vi "Logger_SARAH.vi"() -> ()   [LabVIEW 2017]
uses:
  DefDeType/ListeMachineEtats.ctl
  DefDeType/ClusterRefCtrlUSBB.ctl
  DefDeType/WhichPath.ctl
  <vilib>/DAQmx/write.llb/DAQmx Write (Digital Bool 1Line 1Point).vi
  <vilib>/DAQmx/read.llb/DAQmx Read (Analog 1D Wfm NChan NSamp).vi
  <vilib>/DAQmx/create/channels.llb/DAQmx Create Channel (DO-Digital Output).vi
  <vilib>/DAQmx/miscellaneous.llb/DAQmx Fill In Error Info.vi
  <vilib>/DAQmx/configure/task.llb/DAQmx Configure Logging (TDMS).vi
  <vilib>/DAQmx/configure/trigger.llb/DAQmx Start Trigger (Digital Edge).vi
panel:
  in  "Tempo Mes-Largage (ms)":i32=1000
  in  "Tempo Houle - Mes (ms)":i32=5000
  in  "Reprocess":bool
  in  "Calibration":bool
  in  "NextTest Num":u32
  out "num iteration":i32
  out "Acquisition Time":dbl(slide) max=10.0 scale=0.0..1000.0
  in  "ModifConfig":bool
  out "Test List":i32(listbox)=-1
  in  "Bouton Stop":bool
  in  "Bouton Rec":bool
  out "Projet :":string
  out "message":string
  in  "Bouton Quit":bool
  out "LoopTime":u32(graph)
  out "Graph1":waveform(dbl)[](graph)
  # "Data Logger"
  # "Actions"
  # "Project"
  # "PCI Channels"
  # "Test List"
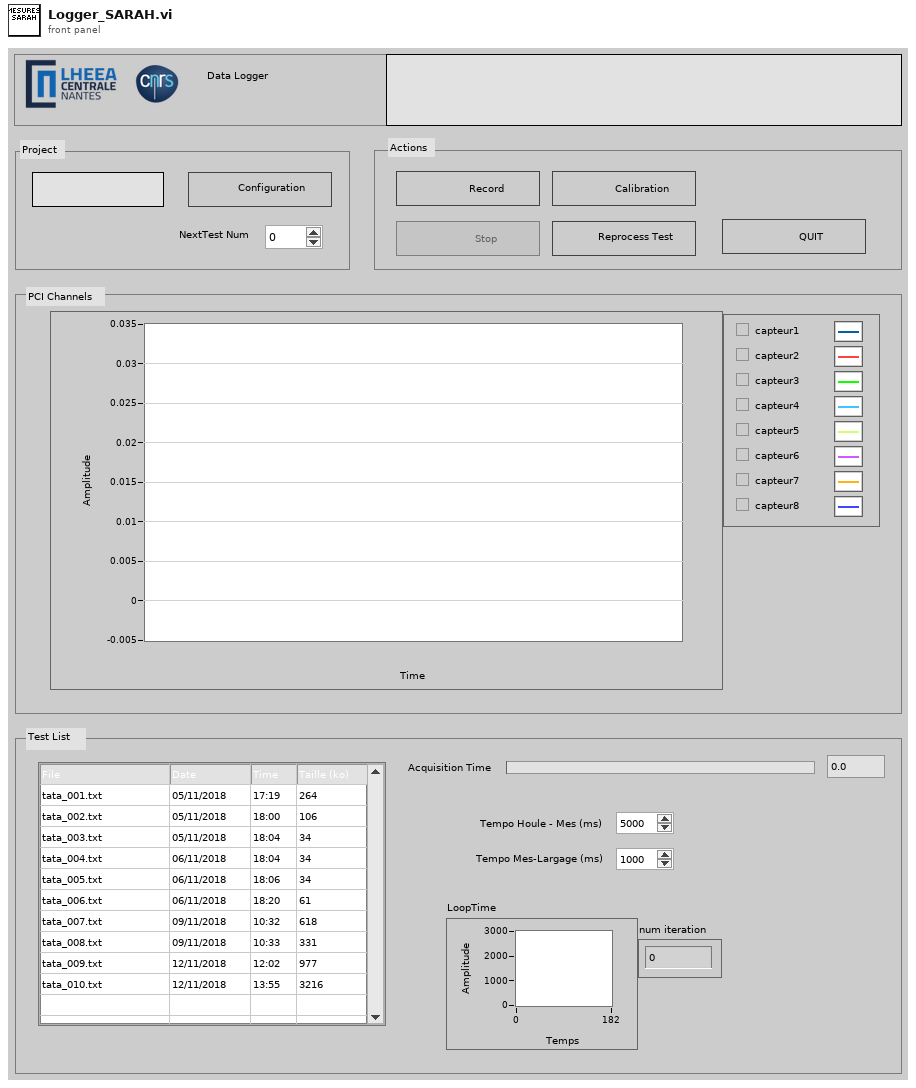
[diagram p1: front panel]
types:
  T1 = typedef "ClusterRefCtrlUSBB.ctl" = cluster{"Reprocess":refnum<vi>, "ModifConfig":refnum<vi>, "Bouton Rec":refnum<vi>, "Bouton Stop":refnum<vi>, "Bouton Quit":refnum<vi>, "Calibration":refnum<vi>, "Test List":refnum<vi>, "NextTest Num":refnum<vi>, "message":refnum<vi>}
  T2 = typedef "ListeMachineEtats.ctl" = enum16{"Init", "NewProj", "OpenProj", "InitLect", "Lect", "InitRec", "Rec", "Processing", "Quit"}
  T3 = typedef "WhichPath.ctl" = enum16{"DossierProjet", "Config", "Meas", "MeasPCI", "MeasCRIO1", "MeasCRIO2", "MeasQualisys", "MeasHBM", "MeasTDMS", "Fig", "Res"}
  T4 = enum8{"Enabled", "Disabled", "Disabled and Grayed Out"}
  T5 = enum32{"Invalid", "Standard", "Closed", "Hidden", "Minimized", "Maximized"}
  T6 = cluster{"Graph2Index":i32[], "Graph1Index":i32[]}
  T7 = typedef "ConfigTotale.ctl" = cluster{"VoltageChannels":T8, "WheastoneBridgeChannels":T9, "Configuration":T10}
  T8 = typedef "VoltageChannels.ctl" = cluster{"ChannelNames":string[], "Sensitivity(Unit/V)":dbl[], "AutoZero":bool[], "ChannelUnits":string[], "Offsets(Units)":dbl[], "Graph Num":u8[]}
  T9 = typedef "WBridgeChannels.ctl" = cluster{"ChannelNames":string[], "Sensitivity(Unit/V)":dbl[], "AutoZero":bool[], "ChannelUnits":string[], "Offsets(Units)":dbl[], "Graph Num":u8[]}
  T10 = typedef "Configuration.ctl" = cluster{"AcqSamplingRate(Hz)":u32, "AcqTime(s)":u32, "Trigger":bool, "NbVoltageChannels":u32, "NbWBridgeChannels":u32, "Qualisys":bool, "Hexapode":bool, "FinalSamplingRate(Hz)":u32, "QualisysDataType":enum16{"6DOF", "3DTracking", "6DOF + 3D"}, "Nortek":bool, "HBM":bool}
  T11 = cluster{"Acquisition Time":refnum<vi>, "Graph1":refnum<vi>}
  T12 = typedef "MergeFileConfig.ctl" = cluster{"Test Num : ":u32, "Project :":string, "Qualisys file":path, "HBM file":path, "QualisysDataType":enum16{"6DOF", "3DTracking", "6DOF + 3D"}, "Qualisys":bool, "HBM":bool}
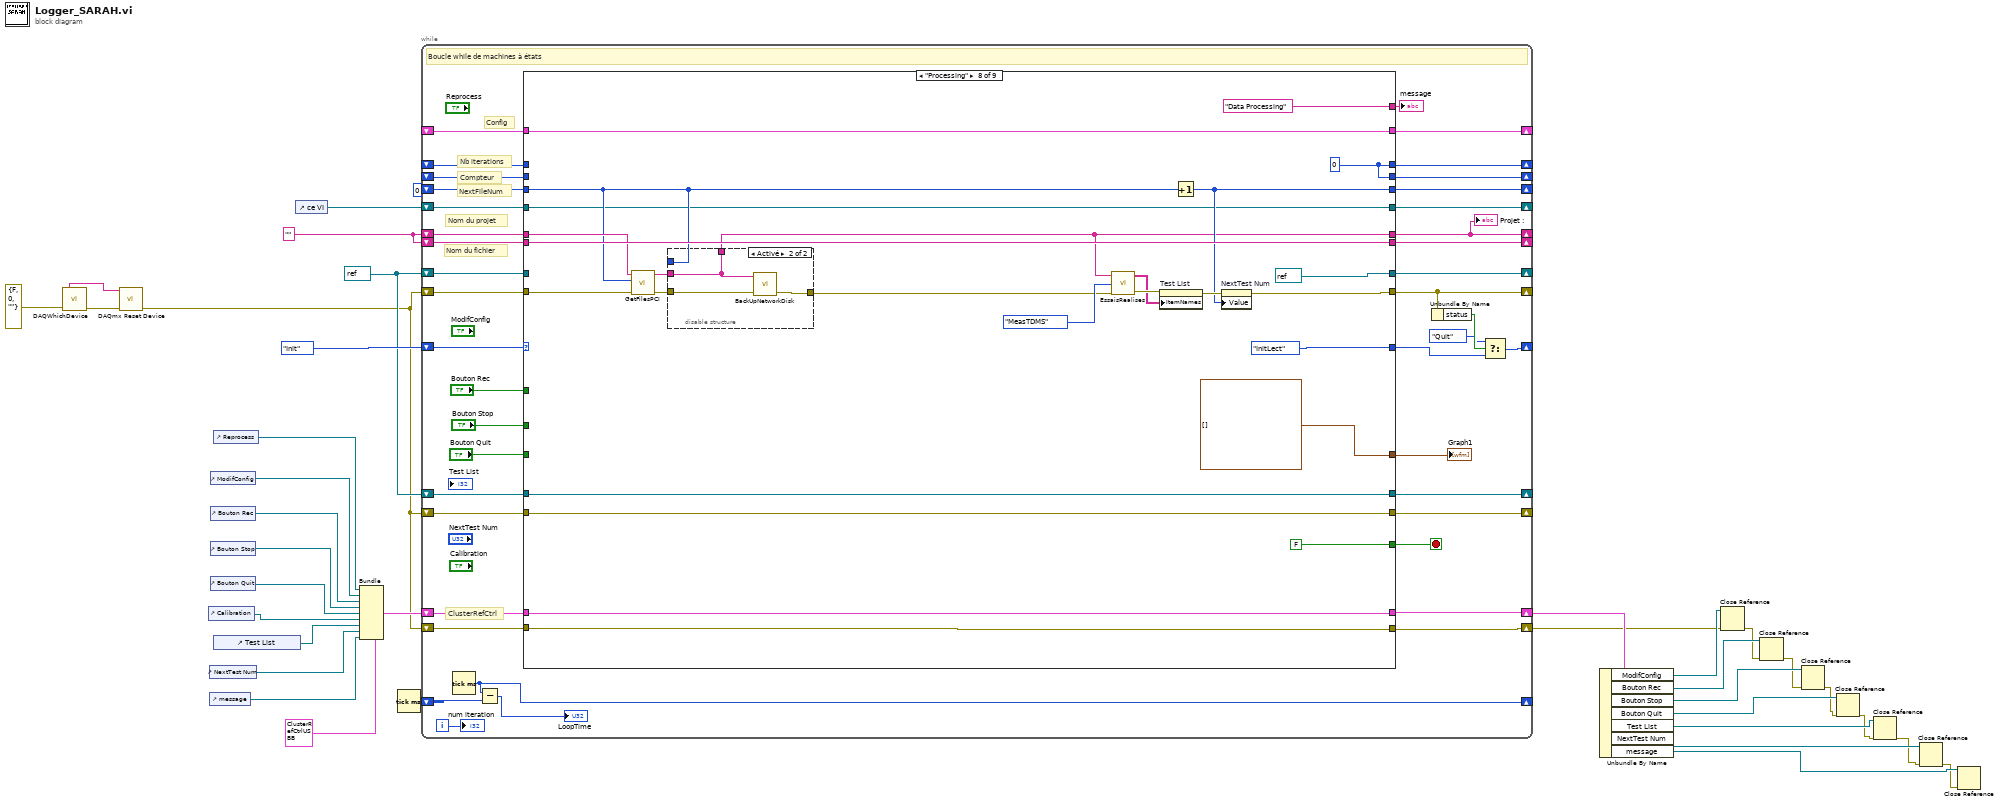
[diagram p0: block diagram]
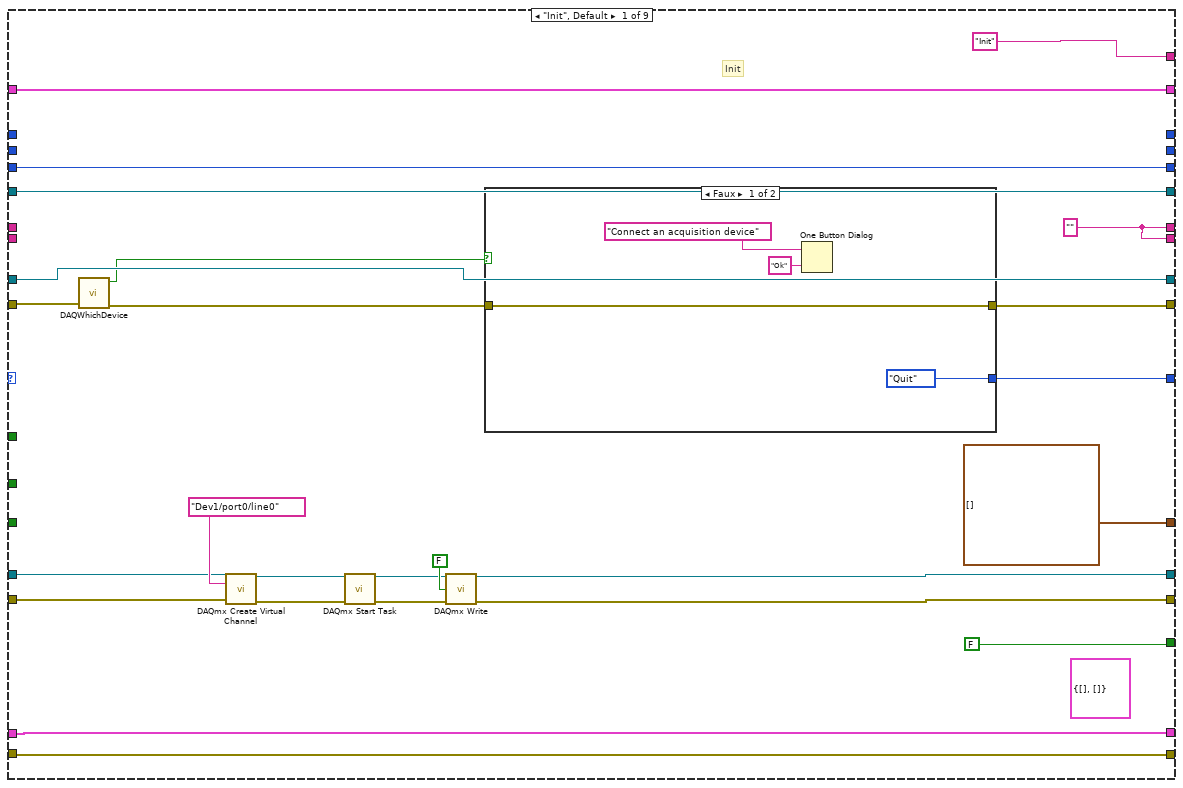
[diagram p2: hidden frame]
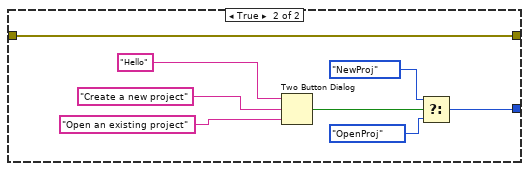
[diagram p3: hidden frame]
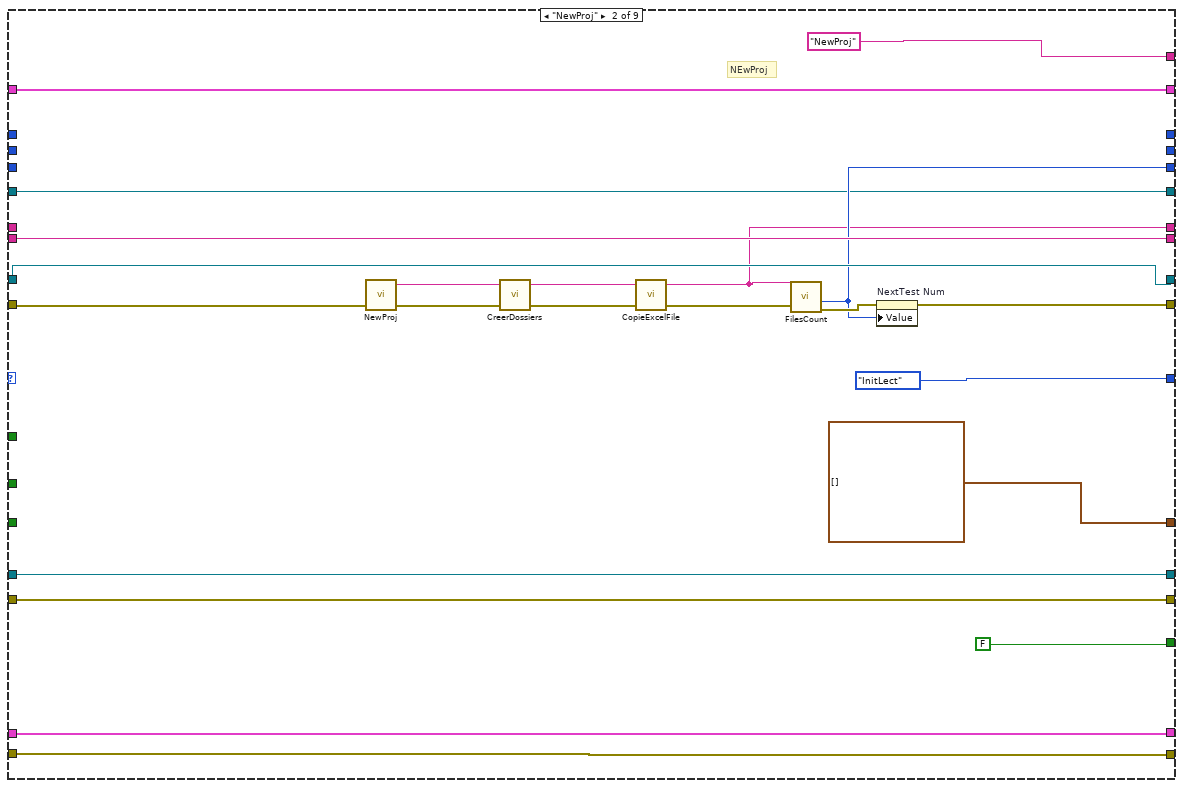
[diagram p4: hidden frame]
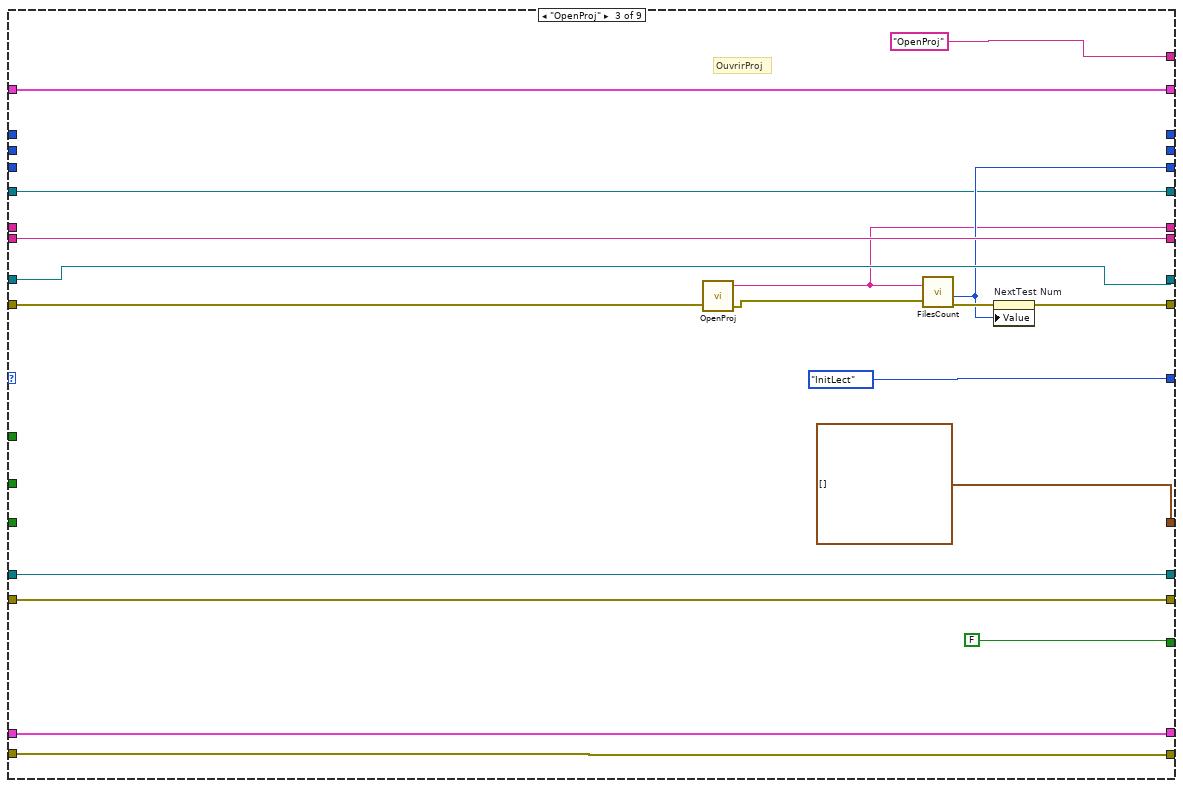
[diagram p5: hidden frame]
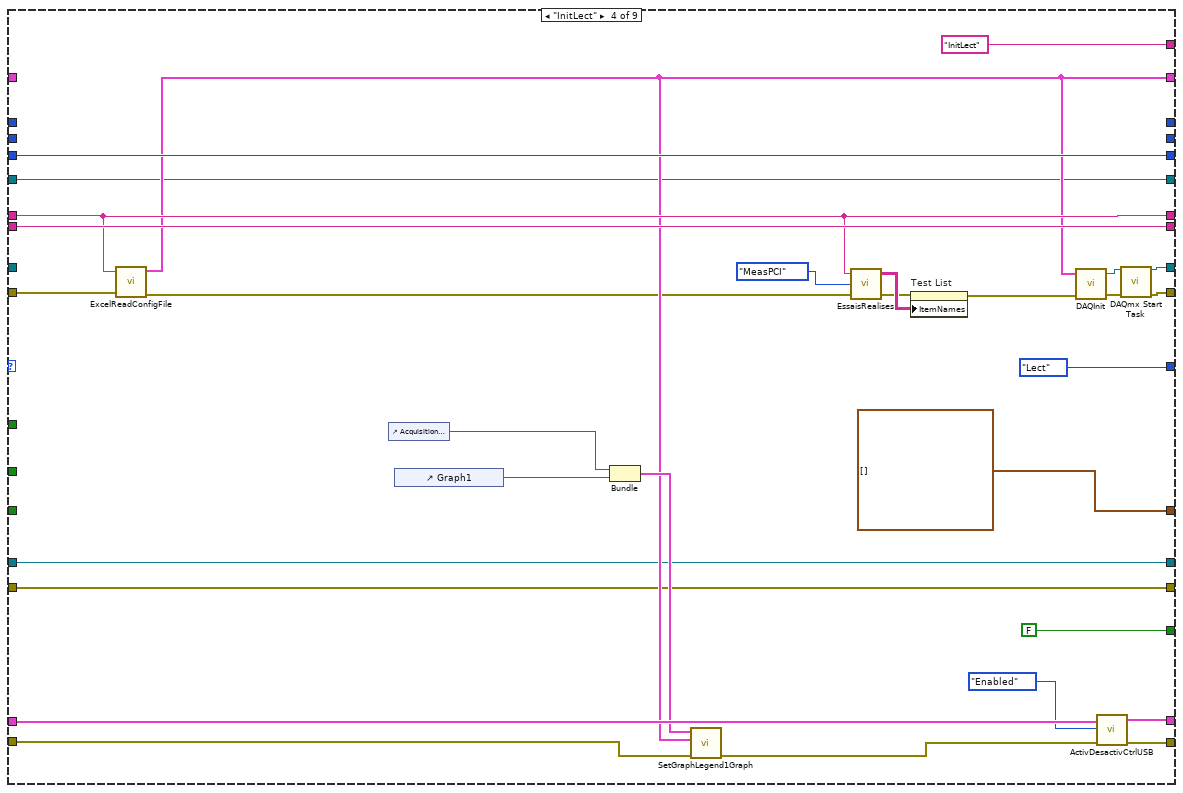
[diagram p6: hidden frame]
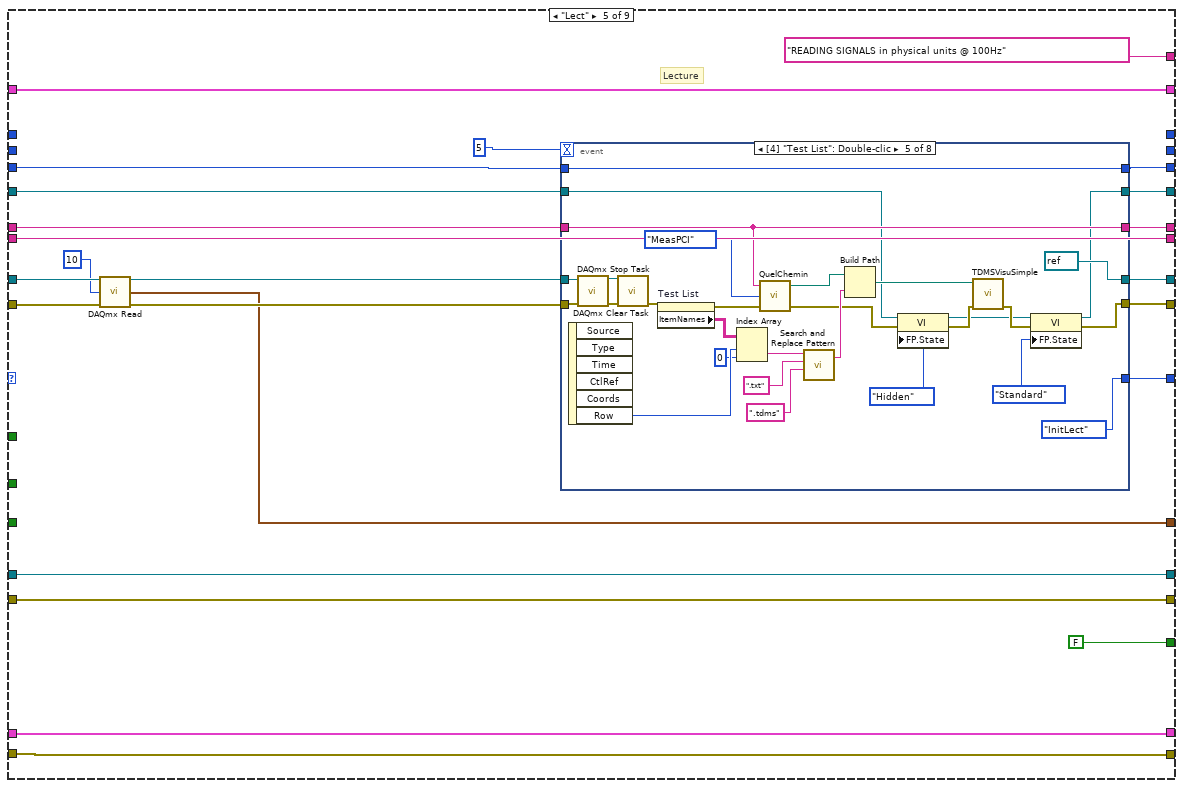
[diagram p7: hidden frame]
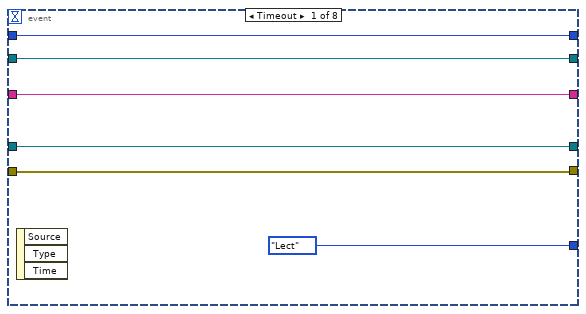
[diagram p8: hidden frame]
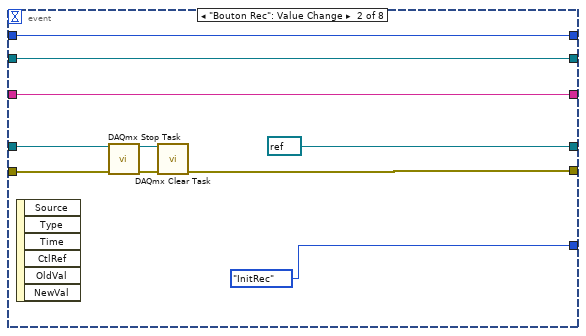
[diagram p9: hidden frame]
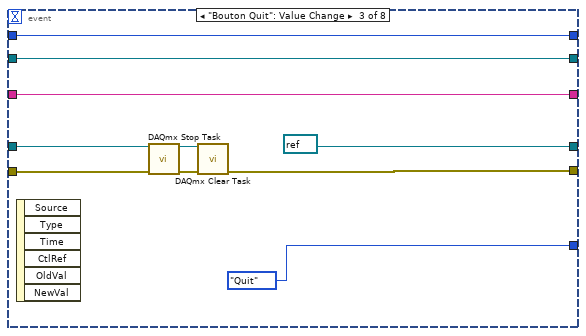
[diagram p10: hidden frame]
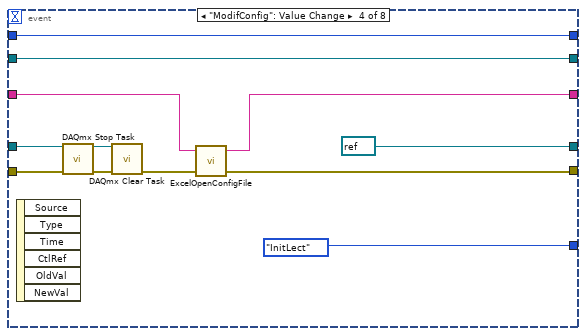
[diagram p11: hidden frame]
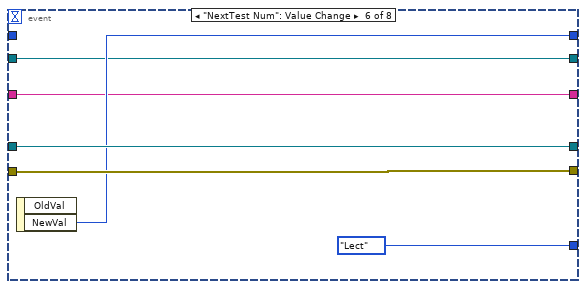
[diagram p12: hidden frame]
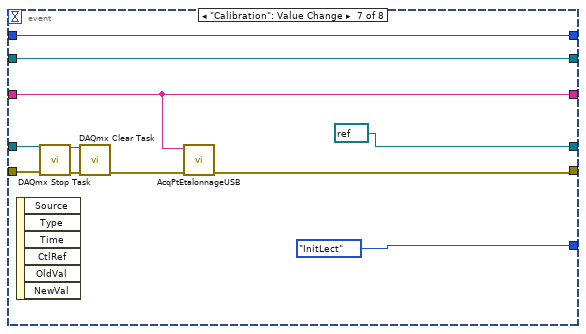
[diagram p13: hidden frame]
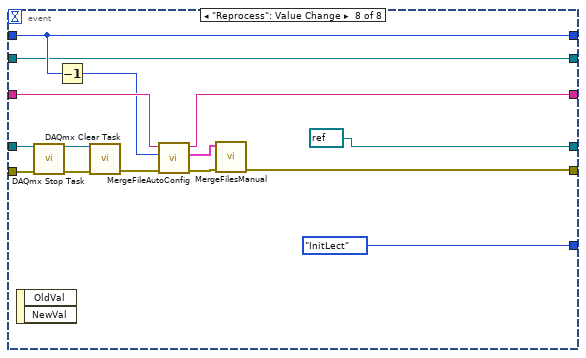
[diagram p14: hidden frame]
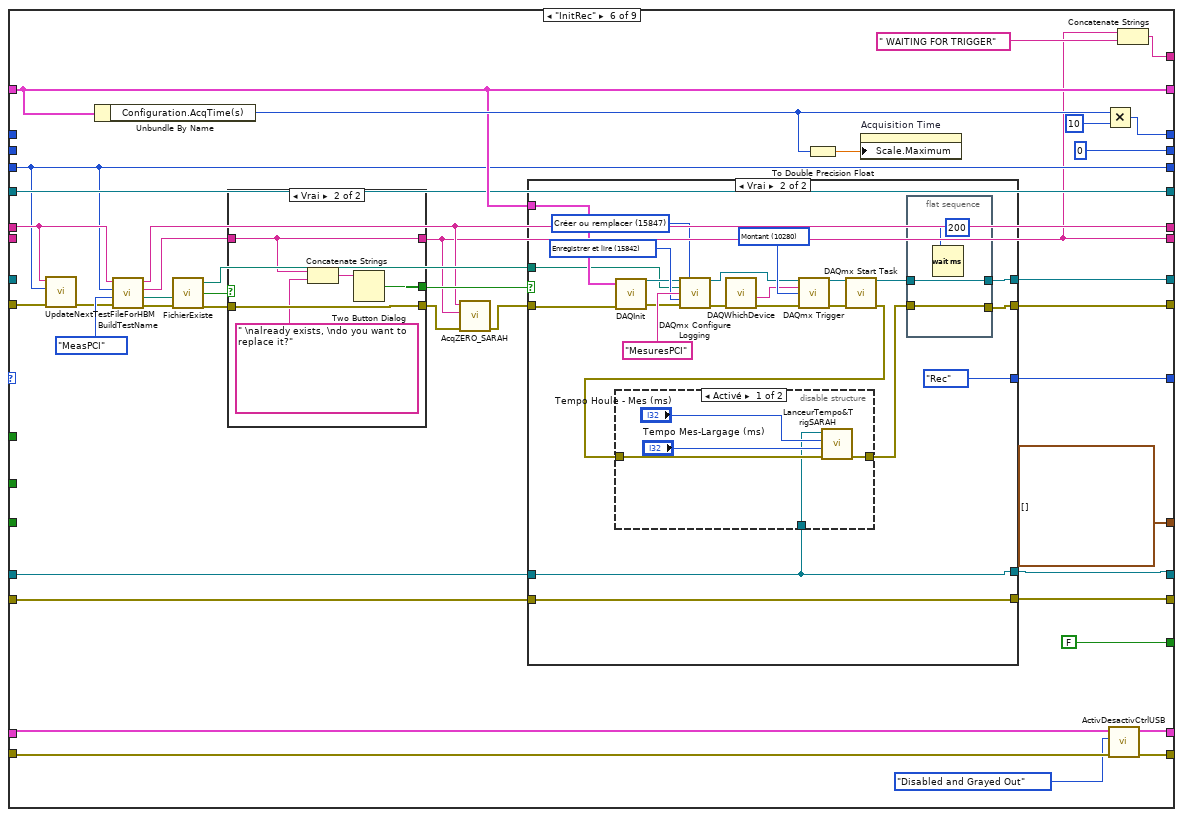
[diagram p15: hidden frame]
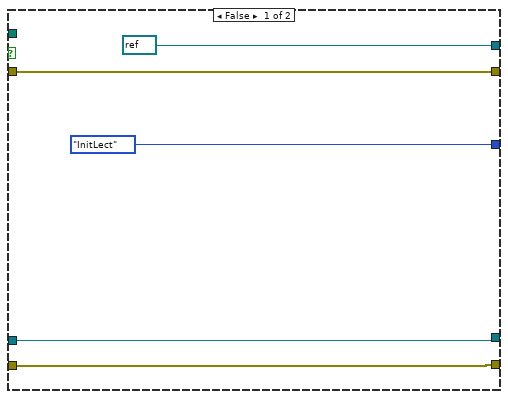
[diagram p16: hidden frame]
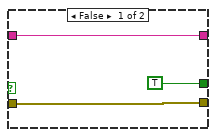
[diagram p18: hidden frame]
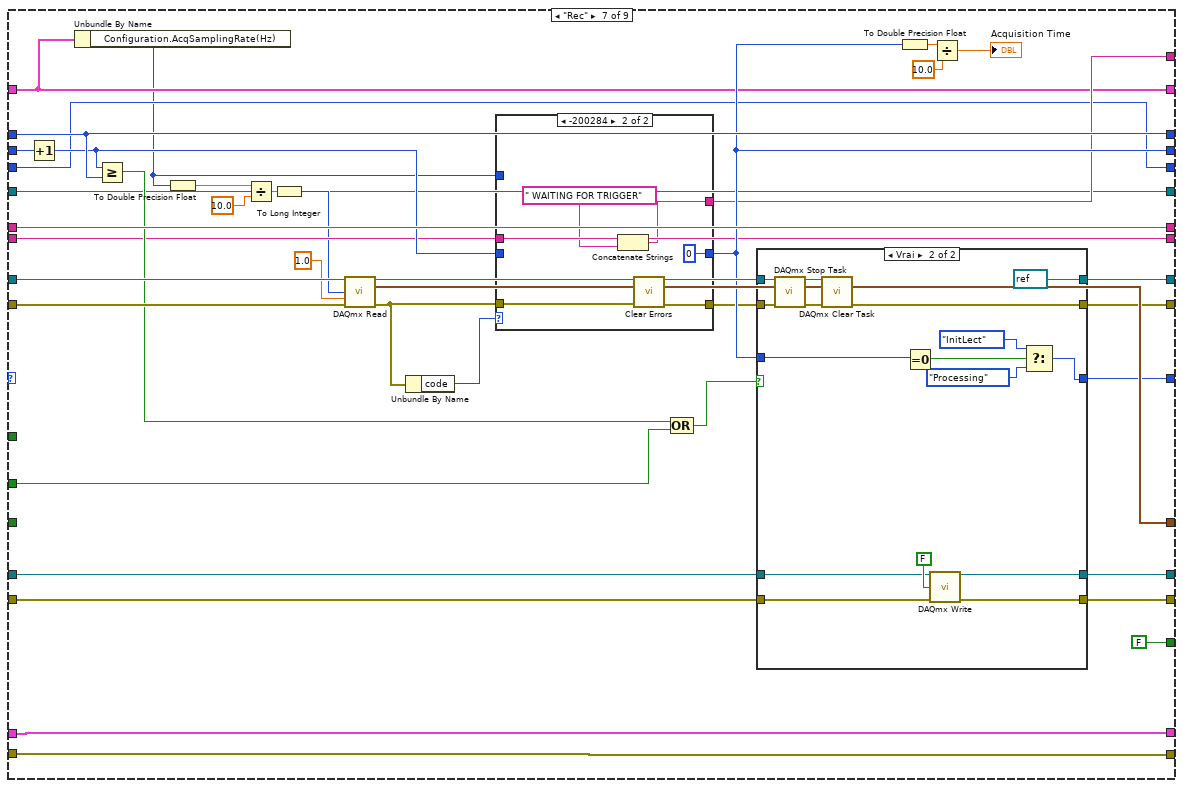
[diagram p19: hidden frame]
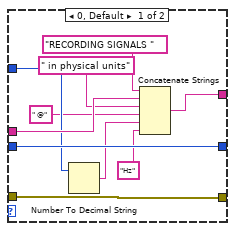
[diagram p20: hidden frame]
diagram:
  w33 = "" ("NomProjetOUT")
  w5 = refnum<k21> refnum ("task out")
  n1 = call "DAQWhichDevice.vi"("error in"=errorcluster {"status"=FALSE, "code"=0, "source"=""} ("error out")) -> ("error out"=w3:errorcluster, "Nom de périphérique DAQmx classique"=w1:tag)  [unwired: 1 in, 5 out]
  n2 = call <vilib>:"DAQmx Reset Device.vi"("device in"=w1, "error in"=w3) -> ("error out"=w2:errorcluster)  [unwired: 13 in]
  n3 = control-ref of="Calibration"() -> (w10:refnum<vi>)
  n4 = control-ref of="NextTest Num"() -> (w27:refnum<vi>)
  n5 = control-ref of="message"() -> (w26:refnum<vi>)
  n6 = control-ref of="ModifConfig"() -> (w32:refnum<vi>)
  n7 = control-ref of="Bouton Rec"() -> (w31:refnum<vi>)
  n8 = control-ref of="Bouton Stop"() -> (w30:refnum<vi>)
  n9 = control-ref of="Bouton Quit"() -> (w29:refnum<vi>)
  n10 = control-ref of="Reprocess"() -> (w9:refnum<vi>)
  n11 = control-ref of="Test List"() -> (w28:refnum<vi>)
  n12 = control-ref of="ce VI"() -> (w6:refnum<vi>)
  n13 = Bundle(cluster=T1 {"Reprocess"=refnum, "ModifConfig"=refnum, "Bouton Rec"=refnum, "Bouton Stop"=refnum, "Bouton Quit"=refnum, "Calibration"=refnum, "Test List"=refnum, "NextTest Num"=refnum, "message"=refnum} ("ClusterRefCtrl"), "Reprocess"=w9, "ModifConfig"=w32, "Bouton Rec"=w31, "Bouton Stop"=w30, "Bouton Quit"=w29, "Calibration"=w10, "Test List"=w28, "NextTest Num"=w27, "message"=w26) -> (w7:T1)
  n14 = Tick Count (ms)() -> (millisecond timer value=w36:u32)
  n15 = while {
    shift-right: [w46] -> _
    shift-left: ListeMachineEtats."Init" ("ListeMachineEtats") -> [w61]
    shift-right: [w52] -> _
    shift-left: w33 -> [w76]
    shift-right: [w45] -> _
    shift-left: w2 -> [w75]
    shift-right: [w74] -> _
    shift-left: w5 -> [w73]
    shift-right: [w68] -> _
    shift-left: w33 -> [w67]
    shift-right: [w65] -> _
    shift-left: w36 -> [w66]
    shift-right: [w63] -> _
    shift-left: _ -> [w62]
    shift-right: [w41] -> w17
    shift-left: w2 -> [w60]
    shift-right: [w59] -> _
    shift-left: _ -> [w58]
    shift-right: [w57] -> _
    shift-left: _ -> [w56]
    shift-right: [w54] -> _
    shift-left: u32 0 ("NewVal") -> [w53]
    shift-right: [w50] -> w25
    shift-left: w7 -> [w51]
    shift-right: [w43] -> _
    shift-left: w6 -> [w44]
    shift-right: [w37] -> _
    shift-left: w2 -> [w40]
    shift-right: [w38] -> _
    shift-left: w5 -> [w39]
    i -> [w55]
    stop <- w72 stop-if-true
    # "ClusterRefCtrl"
    # "NextFileNum"
    # "Compteur"
    # "Nb iterations"
    # "Config"
    # "Nom du fichier"
    # "Nom du projet"
    # "Boucle while de machines à états"
    n16 = Tick Count (ms)() -> (millisecond timer value=w65:u32)
    n17 = Subtract(x=w65, y=w66) -> (x-y=→"LoopTime":u32)
    n18 = case shown="\"Processing\"" w61 {
      tunnel: [w102 ListeMachineEtats."InitLect" ("ListeMachineEtats") ListeMachineEtats."InitLect" ("ListeMachineEtats") ListeMachineEtats."Lect" ("ListeMachineEtats") w198 w338 w423 ListeMachineEtats."InitLect" ("ListeMachineEtats") ListeMachineEtats."Init" ("ListeMachineEtats")] -> w48
      tunnel: ["Init" ("message") "NewProj" ("message") "OpenProj" ("message") "InitLect" ("message") "READING SIGNALS in physical units @ 100Hz" ("message") w337 w404 "Data Processing" ("message") "Quitter" ("message")] -> w77
      tunnel: [w92 w119 w141 w170 w191 w309 w422 w475 w525] -> w52
      tunnel: w76 -> [_ _ _ w170 w197 w317 w422 w478 _]
      tunnel: [w95 w122 w143 w177 w200 w343 w424 w483 w511] -> w45
      tunnel: w75 -> [w97 w131 w153 w171 w206 w319 w430 w479 w517]
      tunnel: [w100 w130 w152 w179 w199 w344 w425 refnum<k21> refnum ("task out") w504] -> w74
      tunnel: w73 -> [w100 w130 w152 _ w207 _ w429 _ w516]
      tunnel: [waveform(dbl)[] [] ("data") waveform(dbl)[] [] ("data") waveform(dbl)[] [] ("data") waveform(dbl)[] [] ("data") w190 waveform(dbl)[] [] ("data") w428 waveform(dbl)[] [] ("data") waveform(dbl)[] [] ("data")] -> w42
      tunnel: [FALSE FALSE FALSE FALSE FALSE FALSE FALSE FALSE TRUE] -> w72
      tunnel: "Bouton Quit" -> [_ _ _ _ _ _ _ _ _]
      tunnel: "Bouton Rec" -> [_ _ _ _ _ _ _ _ _]
      tunnel: "Bouton Stop" -> [_ _ _ _ _ _ w421 _ _]
      tunnel: [w92 w127 w149 w176 w203 w308 w405 w489 w525] -> w68
      tunnel: w67 -> [_ w127 w149 w176 w203 _ w405 w489 _]
      tunnel: [w94 w126 w148 w160 w195 w328 w400 w486 w524] -> w63
      tunnel: w62 -> [w94 w126 w148 _ w195 w328 w400 w486 w524]
      tunnel: w60 -> [w93 w125 w147 w163 w196 w326 w419 w488 w523]
      tunnel: [w93 w125 w147 w169 w196 w327 w419 w488 w523] -> w41
      tunnel: [_ _ _ _ _ w340 w415 w480 w521] -> w59
      tunnel: w58 -> [_ _ _ _ _ _ w415 _ _]
      tunnel: [_ _ _ _ _ u32 0 ("y") w408 w480 w521] -> w57
      tunnel: w56 -> [_ _ _ _ _ _ w398 _ _]
      tunnel: [w90 w121 w142 w174 w194 w316 w403 w482 w521] -> w54
      tunnel: w53 -> [w90 _ _ w174 w193 w316 w403 w473 _]
      tunnel: w51 -> [w91 w118 w140 w168 w189 w323 w397 w471 w520]
      tunnel: [w91 w118 w140 w167 w189 w324 w397 w471 w520] -> w50
      tunnel: w44 -> [w89 w117 w139 w159 w188 w321 w396 w470 w513]
      tunnel: [w89 w117 w139 w159 w187 w321 w396 w470 w510] -> w43
      tunnel: w40 -> [w85 w116 w138 w156 w185 w315 w395 w469 w507]
      tunnel: [w84 w116 w138 w156 w185 w314 w394 w469 w505] -> w37
      tunnel: [w83 w115 w137 w157 w186 w312 w392 w468 w504] -> w38
      tunnel: w39 -> [w78 w115 w137 w157 w186 w313 w393 w468 w506]
      frame "Init", Default {
        (unwired) T6 {"Graph2Index"=[], "Graph1Index"=[]} ("GraphIndex")
        w92 = "" ("NomProjet")
        # "Init"
        n19 = call "DAQWhichDevice.vi"("error in"=w97) -> ("error out"=w86:errorcluster, "OK?"=w96:bool)  [unwired: 1 in, 5 out]
        n20 = call-poly <vilib>:"DAQmx Create Virtual Channel.vi"("task in"=w78, "lines"=tag "Dev1/port0/line0", "error in"=w85) -> ("task out"=w82:refnum<k21>, "error out"=w81:errorcluster)  [unwired: 11 in]
        n21 = call <vilib>:"DAQmx Start Task.vi"("task/channels in"=w82, "error in"=w81) -> ("task out"=w80:refnum<k21>, "error out"=w79:errorcluster)  [unwired: 12 in]
        n22 = call-poly <vilib>:"DAQmx Write.vi"("task/channels in"=w80, "data"=FALSE, "error in"=w79) -> ("task out"=w83:refnum<k21>, "error out"=w84:errorcluster)  [unwired: 10 in, 1 out]
        n23 = case shown="Faux" w96 {
          tunnel: [ListeMachineEtats."Quit" ("ListeMachineEtats") w110] -> w102
          tunnel: w86 -> [w106 w109]
          tunnel: [w106 w109] -> w95
          frame False {
            n24 = One Button Dialog(message="Connect an acquisition device", button name ("OK")="Ok" ("nom du bouton (\"OK\")")) -> ()  [unwired: 1 out]
          }
          frame True {
            n25 = Two Button Dialog(message="Hello", 1:"Open an existing project" ("Nom du bouton F (\"Annuler\")"), 2:"Create a new project" ("Nom du bouton V (\"OK\")")) -> (T button?=w111:bool)
            n26 = Select(t=ListeMachineEtats."NewProj" ("ListeMachineEtats"), s=w111, f=ListeMachineEtats."OpenProj" ("ListeMachineEtats")) -> (s? t:f=w110:T2)
          }
        }
      }
      frame "NewProj" {
        # "NEwProj"
        n27 = call "NewProj.vi"("entrée d'erreur"=w131) -> ("sortie d'erreur"=w134:errorcluster, "NomProjet"=w135:string)  [unwired: 3 in]
        n28 = call "CreerDossiers.vi"("Entrée d'erreur"=w134, "NomProjet"=w135) -> ("error out"=w133:errorcluster, "NomProjetOut"=w132:string)  [unwired: 2 in]
        n29 = call "CopieExcelFile.vi"("Entrée d'erreur"=w133, "NomProjet"=w132) -> ("sortie d'erreur"=w120:errorcluster, "NomProjetOut"=w119:string)  [unwired: 2 in]
        n30 = call "FilesCount.vi"("NomProjet"=w119, "entrée d'erreur"=w120) -> ("NextTestNum"=w121:u32, "sortie d'erreur"=w123:errorcluster)  [unwired: 4 out]
        n31 = property on="NextTest Num" class="NumNb (strict)"(error in=w123, "Value"=w121) -> (error out=w122:errorcluster)  [unwired: 1 in, 1 out]
      }
      frame "OpenProj" {
        # "OuvrirProj"
        n32 = call "OpenProj.vi"("entrée d'erreur"=w153) -> ("sortie d'erreur"=w145:errorcluster, "NomProjet"=w141:string)  [unwired: 3 in]
        n33 = call "FilesCount.vi"("NomProjet"=w141, "entrée d'erreur"=w145) -> ("NextTestNum"=w142:u32, "sortie d'erreur"=w144:errorcluster)  [unwired: 4 out]
        n34 = property on="NextTest Num" class="NumNb (strict)"(error in=w144, "Value"=w142) -> (error out=w143:errorcluster)  [unwired: 1 in, 1 out]
      }
      frame "InitLect" {
        n35 = call "ExcelReadConfigFile.vi"("NomProjet"=w170, "error in (no error)"=w171) -> ("ConfigurationTotale"=w160:T7, "error out"=w158:errorcluster)  [unwired: 3 in]
        n36 = control-ref of="Acquisition Time"() -> (w165:refnum<vi>)
        n37 = control-ref of="Graph1"() -> (w164:refnum<vi>)
        n38 = Bundle("Acquisition Time"=w165, "Graph1"=w164) -> (w161:T11)  [unwired: 1 in]
        n39 = call "SetGraphLegend1Graph.vi"("error in (no error)"=w163, "ConfigTotale"=w160, "ClusterRefGraphs"=w161) -> ("error out"=w162:errorcluster)  [unwired: 4 in]
        n40 = call "EssaisRealises.vi"("entrée d'erreur (pas d'erreur)"=w158, "WhichPath?"=WhichPath."MeasPCI", "NomProjet"=w170) -> ("sortie d'erreur"=w172:errorcluster, "InfosFichiers"=w173:string[][])  [unwired: 1 in]
        n41 = property on="Test List" class="ListeMCol (strict)"(error in=w172, "ItemNames"=w173) -> (error out=w181:errorcluster)  [unwired: 1 in, 1 out]
        n42 = call "DAQInit.vi"("error in"=w181, "configInput"=w160) -> ("error out"=w178:errorcluster, "task out"=w180:refnum<k21>)  [unwired: 2 in]
        n43 = call "ActivDesactivCtrlUSB.vi"("error in (no error)"=w162, "Disabled"=T4."Enabled", "ClusterRefCtrl_IN"=w168) -> ("error out"=w169:errorcluster, "ClusterRefCtrl_OUT"=w167:T1)  [unwired: 3 in]
        n44 = call <vilib>:"DAQmx Start Task.vi"("task/channels in"=w180, "error in"=w178) -> ("task out"=w179:refnum<k21>, "error out"=w177:errorcluster)  [unwired: 12 in]
      }
      frame "Lect" {
        # "Lecture"
        n45 = call-poly <vilib>:"DAQmx Read.vi"("task/channels in"=w207, "number of samples per channel"=10, "error in"=w206) -> ("task out"=w202:refnum<k21>, "data"=w190:waveform(dbl)[], "error out"=w192:errorcluster)  [unwired: 10 in]
        n46 = event shown="[4] \"Test List\": Double-clic" {
          selector: _ -> [_ _ _ _ _ _ _ _]
          dyn-events: _ -> [_ _ _ _ _ _ _ _]
          timeout: 5 -> [_ _ _ _ _ _ _ _]
          tunnel: w192 -> [w214 w222 w232 w243 w262 w280 w290 w302]
          tunnel: w202 -> [w213 w221 w231 w244 w265 w281 w291 w303]
          tunnel: [w214 w220 w230 w240 w250 w280 w284 w295] -> w200
          tunnel: [w213 refnum<k21> refnum ("task out") refnum<k21> refnum ("task out") refnum<k21> refnum ("task out") refnum<k21> refnum ("task out") w281 refnum<k21> refnum ("task out") refnum<k21> refnum ("task out")] -> w199
          tunnel: [ListeMachineEtats."Lect" ("ListeMachineEtats") ListeMachineEtats."InitRec" ("ListeMachineEtats") ListeMachineEtats."Quit" ("ListeMachineEtats") ListeMachineEtats."InitLect" ("ListeMachineEtats") ListeMachineEtats."InitLect" ("ListeMachineEtats") ListeMachineEtats."Lect" ("ListeMachineEtats") ListeMachineEtats."InitLect" ("ListeMachineEtats") ListeMachineEtats."InitLect" ("ListeMachineEtats")] -> w198
          tunnel: w197 -> [w210 w216 w226 w239 w259 w277 w285 w301]
          tunnel: [w211 w217 w227 w237 w260 w278 w283 w294] -> w194
          tunnel: w193 -> [w211 w217 w227 w237 w260 _ w283 w294]
          tunnel: [w210 w216 w226 w236 w259 w277 w285 w296] -> w191
          tunnel: w188 -> [w209 w215 w225 w235 w253 w276 w282 w293]
          tunnel: [w209 w215 w225 w235 w247 w276 w282 w293] -> w187
          event Timeout {
            n47 = event-data() -> ()  [unwired: 1 in, 3 out]
          }
          event "Bouton Rec": Value Change {
            n48 = event-data() -> ()  [unwired: 1 in, 6 out]
            n49 = call <vilib>:"DAQmx Stop Task.vi"("task/channels in"=w221, "error in"=w222) -> ("task out"=w223:refnum<k21>, "error out"=w224:errorcluster)  [unwired: 12 in]
            n50 = call <vilib>:"DAQmx Clear Task.vi"("task in"=w223, "error in"=w224) -> ("error out"=w220:errorcluster)  [unwired: 13 in]
          }
          event "Bouton Quit": Value Change {
            n51 = event-data() -> ()  [unwired: 1 in, 6 out]
            n52 = call <vilib>:"DAQmx Stop Task.vi"("task/channels in"=w231, "error in"=w232) -> ("task out"=w233:refnum<k21>, "error out"=w234:errorcluster)  [unwired: 12 in]
            n53 = call <vilib>:"DAQmx Clear Task.vi"("task in"=w233, "error in"=w234) -> ("error out"=w230:errorcluster)  [unwired: 13 in]
          }
          event "ModifConfig": Value Change {
            n54 = event-data() -> ()  [unwired: 1 in, 6 out]
            n55 = call <vilib>:"DAQmx Stop Task.vi"("task/channels in"=w244, "error in"=w243) -> ("task out"=w245:refnum<k21>, "error out"=w246:errorcluster)  [unwired: 12 in]
            n56 = call <vilib>:"DAQmx Clear Task.vi"("task in"=w245, "error in"=w246) -> ("error out"=w241:errorcluster)  [unwired: 13 in]
            n57 = call "ExcelOpenConfigFile.vi"("error in (no error)"=w241, "NomProjet"=w239) -> ("sortie d'erreur"=w240:errorcluster, "NomProjetOut"=w236:string)  [unwired: 2 in]
          }
          event "Test List": Double Click {
            n58 = event-data() -> ("Row"=w274:i32)  [unwired: 1 in, 5 out]
            n59 = call <vilib>:"DAQmx Stop Task.vi"("task/channels in"=w265, "error in"=w262) -> ("task out"=w264:refnum<k21>, "error out"=w263:errorcluster)  [unwired: 12 in]
            n60 = call <vilib>:"DAQmx Clear Task.vi"("task in"=w264, "error in"=w263) -> ("error out"=w266:errorcluster)  [unwired: 13 in]
            n61 = property on="Test List" class="ListeMCol (strict)"(error in=w266) -> (error out=w269:errorcluster, "ItemNames"=w275:string[][])  [unwired: 1 in, 1 out]
            n62 = Index Array(array=w275, index (row)=w274, index (col)=0 ("indice désactivé (col)")) -> (element=w270:string)
            n63 = call "QuelChemin.vi"("Entrée d'erreur"=w269, "WhichPath?"=WhichPath."MeasPCI", "NomProjet"=w259) -> ("Sortie d'erreur"=w255:errorcluster, "SurDisqueLocal"=w268:path)  [unwired: 1 out]
            n64 = call <vilib>:"Search and Replace Pattern.vi"("string"=w270, "regular expression (\"\")"=".txt" ("regular expression (\"\")"), "replace string (\"\")"=".tdms" ("replace string (\"\")")) -> ("result string"=w256:string)  [unwired: 2 in, 1 out]
            n65 = Build Path(base path=w268, name or relative path=w256) -> (appended path=w257:path)
            n66 = property class="VI"(reference=w253, error in=w255, "FP.State"=T5."Hidden" ("Fenêtre face-avant:État")) -> (reference out=w248:refnum<vi>, error out=w254:errorcluster)
            n67 = call "TDMSVisuSimple.vi"("entrée d'erreur"=w254, "chemin du fichier"=w257) -> ("sortie d'erreur"=w251:errorcluster)  [unwired: 5 in]
            n68 = property class="VI"(reference=w248, error in=w251, "FP.State"=T5."Standard" ("Fenêtre face-avant:État")) -> (reference out=w247:refnum<vi>, error out=w250:errorcluster)
          }
          event "NextTest Num": Value Change {
            n69 = event-data() -> ("NewVal"=w278:u32)  [unwired: 1 in, 1 out]
          }
          event "Calibration": Value Change {
            n70 = event-data() -> ()  [unwired: 1 in, 6 out]
            n71 = call <vilib>:"DAQmx Stop Task.vi"("task/channels in"=w291, "error in"=w290) -> ("task out"=w292:refnum<k21>, "error out"=w289:errorcluster)  [unwired: 12 in]
            n72 = call <vilib>:"DAQmx Clear Task.vi"("task in"=w292, "error in"=w289) -> ("error out"=w288:errorcluster)  [unwired: 13 in]
            n73 = call "AcqPtEtalonnageUSB.vi"("entrée d'erreur"=w288, "Projet"=w285) -> ("sortie d'erreur"=w284:errorcluster)  [unwired: 5 in]
          }
          event "Reprocess": Value Change {
            n74 = event-data() -> ()  [unwired: 1 in, 2 out]
            n75 = call <vilib>:"DAQmx Stop Task.vi"("task/channels in"=w303, "error in"=w302) -> ("task out"=w305:refnum<k21>, "error out"=w304:errorcluster)  [unwired: 12 in]
            n76 = Decrement(x=w294) -> (x-1=w299:u32)
            n77 = call <vilib>:"DAQmx Clear Task.vi"("task in"=w305, "error in"=w304) -> ("error out"=w300:errorcluster)  [unwired: 13 in]
            n78 = call "MergeFileAutoConfig.vi"("error in (no error)"=w300, "test num"=w299, "ProjetIN"=w301) -> ("error out"=w298:errorcluster, "MergeFileConfigOUT"=w297:T12, "ProjetOUT"=w296:string)  [unwired: 2 in]
            n79 = call "MergeFilesManual.vi"("Error In"=w298, "MergeFileConfINPUT"=w297) -> ("sortie d'erreur"=w295:errorcluster)  [unwired: 5 in]
          }
        }
      }
      frame "InitRec" {
        n80 = call "UpdateNextTestFileForHBM.vi"("entrée d'erreur"=w319, "NextTestNum"=w316, "NomProjet"=w317) -> ("sortie d'erreur"=w318:errorcluster)  [unwired: 4 in]
        n81 = Unbundle By Name(w328) -> ("Configuration.AcqTime(s)"=w331:u32)
        n82 = call "BuildTestName.vi"("entrée d'erreur"=w318, "WhichPath?"=WhichPath."MeasPCI", "NextTestNum"=w316, "NomProjet"=w317) -> ("sortie d'erreur"=w336:errorcluster, "cheminProchainFichier"=w335:path, "NomProchainFichier"=w330:string, "NomProjetOut"=w309:string)  [unwired: 1 in]
        n83 = call "FichierExiste.vi"("entrée d'erreur (pas d'erreur)"=w336, "cheminProchainFichierRAW"=w335) -> ("sortie d'erreur"=w334:errorcluster, "Booléen"=w333:bool, "path out"=w332:path)  [unwired: 1 in]
        n84 = case shown="Vrai" w333 {
          tunnel: [w386 w391] -> w311
          tunnel: w334 -> [w386 w391]
          tunnel: [TRUE ("T button?") w388] -> w329
          tunnel: w330 -> [w384 w387]
          tunnel: [w384 w387] -> w308
          frame False {
          }
          frame True {
            n85 = Concatenate Strings(w387, " \nalready exists, \ndo you want to replace it?" ("chaîne")) -> (w389:string)
            n86 = Two Button Dialog(message=w389) -> (T button?=w388:bool)  [unwired: 2 in]
          }
        }
        n87 = call "AcqZERO_SARAH.vi"("entrée d'erreur"=w311, "Fichier"=w308, "Projet"=w309) -> ("sortie d'erreur"=w310:errorcluster)  [unwired: 4 in]
        n88 = case shown="Vrai" w329 {
          tunnel: [refnum<k21> refnum ("task out") w356] -> w344
          tunnel: [w350 w358] -> w343
          tunnel: [ListeMachineEtats."InitLect" ("ListeMachineEtats") ListeMachineEtats."Rec" ("ListeMachineEtats")] -> w338
          tunnel: w310 -> [w350 w359]
          tunnel: w332 -> [_ w360]
          tunnel: w328 -> [_ w361]
          tunnel: [w347 w353] -> w314
          tunnel: w315 -> [w347 w353]
          tunnel: [w348 w352] -> w312
          tunnel: w313 -> [w348 w352]
          frame False {
          }
          frame True {
            w373 = 10280 items=["Montant"=10280, "Descendant"=10171] ("edge")
            w365 = 15847 items=["Ouvrir"=10437, "Ouvrir ou créer"=15846, "Créer ou remplacer"=15847, "Créer"=15848] ("operation")
            w364 = 15842 items=["Off"=10231, "Enregistrer"=15844, "Enregistrer et lire"=15842] ("logging mode")
            n89 = call "DAQInit.vi"("error in"=w359, "configInput"=w361) -> ("error out"=w362:errorcluster, "task out"=w363:refnum<k21>)  [unwired: 2 in]
            n90 = call-poly <vilib>:"DAQmx Configure Logging.vi"("task/channels in"=w363, "operation"=w365, "file path"=w360, "group name"="MesuresPCI", "logging mode"=w364, "error in"=w362) -> ("task out"=w367:refnum<k21>, "error out"=w366:errorcluster)  [unwired: 8 in]
            n91 = call "DAQWhichDevice.vi"("error in"=w366) -> ("error out"=w371:errorcluster, "sourceTrig"=w372:tag)  [unwired: 1 in, 5 out]
            n92 = call-poly <vilib>:"DAQmx Trigger.vi"("task/channels in"=w367, "source"=w372, "edge"=w373, "error in"=w371) -> ("task out"=w369:refnum<k21>, "error out"=w368:errorcluster)  [unwired: 10 in]
            n93 = call <vilib>:"DAQmx Start Task.vi"("task/channels in"=w369, "error in"=w368) -> ("task out"=w357:refnum<k21>, "error out"=w355:errorcluster)  [unwired: 12 in]
            n94 = disable-structure shown="Activé" {
              disable-tunnel: w355 -> [w379 w380]
              disable-tunnel: [w378 w380] -> w354
              disable-tunnel: w352 -> [w375 _]
              frame Enabled {
                n95 = call "LanceurTempo&TrigSARAH.vi"("entrée d'erreur (pas d'erreur)"=w379, "Tempo Mes-Largage (ms)"="Tempo Mes-Largage (ms)", "Tempo Houle - Mes (ms)"="Tempo Houle - Mes (ms)", "task in"=w375) -> ("sortie d'erreur"=w378:errorcluster)  [unwired: 3 in]
              }
              frame Disabled {
              }
            }
            n96 = flat-sequence {
              tunnel: [w381] -> w358
              tunnel: [w383] -> w356
              tunnel: w357 -> [w383]
              tunnel: w354 -> [w381]
              frame #0 {
                n97 = Wait (ms)(milliseconds to wait=u32 200 ("attente (ms)")) -> ()  [unwired: 1 out]
              }
            }
          }
        }
        n98 = To Double Precision Float(number=w331) -> (double precision float=w342:dbl)
        n99 = property on="Acquisition Time" class="Gliss (strict)"("Scale.Maximum"=w342) -> ()  [unwired: 2 in, 2 out]
        n100 = Multiply(x=w331, y=u32 10) -> (x*y=w340:u32)
        n101 = call "ActivDesactivCtrlUSB.vi"("error in (no error)"=w326, "Disabled"=T4."Disabled and Grayed Out", "ClusterRefCtrl_IN"=w323) -> ("error out"=w327:errorcluster, "ClusterRefCtrl_OUT"=w324:T1)  [unwired: 3 in]
        n102 = Concatenate Strings(w308, " WAITING FOR TRIGGER" ("message")) -> (w337:string)
      }
      frame "Rec" {
        n103 = Increment(x=w398) -> (x+1=w409:u32)
        n104 = Unbundle By Name(w400) -> ("Configuration.AcqSamplingRate(Hz)"=w399:u32)
        n105 = Greater Or Equal?(x=w409, y=w415) -> (x >= y?=w416:bool)
        n106 = To Double Precision Float(number=w399) -> (double precision float=w417:dbl)
        n107 = Divide(x=w417, y=10.0) -> (x/y=w402:dbl)
        n108 = To Long Integer(number=w402) -> (32bit integer=w401:i32)
        n109 = call-poly <vilib>:"DAQmx Read.vi"("task/channels in"=w429, "number of samples per channel"=w401, "timeout"=1.0, "error in"=w430) -> ("task out"=w426:refnum<k21>, "data"=w428:waveform(dbl)[], "error out"=w407:errorcluster)  [unwired: 9 in]
        n110 = Unbundle By Name(w407) -> ("code"=w410:i32)
        n111 = case shown="-200284" w410 {
          tunnel: w409 -> [w440 _]
          tunnel: [w440 u32 0] -> w408
          tunnel: w407 -> [w439 w445]
          tunnel: [w439 w444] -> w406
          tunnel: w405 -> [w437 w443]
          tunnel: [w436 w442] -> w404
          tunnel: w399 -> [w434 _]
          frame 0, Default {
            n112 = Number To Decimal String(number=w434) -> (decimal integer string=w432:string)  [unwired: 1 in]
            n113 = Concatenate Strings("RECORDING SIGNALS " ("message"), w437, " in physical units" ("message"), " @" ("chaîne"), w432, "Hz" ("chaîne")) -> (w436:string)
          }
          frame -200284 {
            n114 = Concatenate Strings(w443, " WAITING FOR TRIGGER" ("message")) -> (w442:string)
            n115 = call <vilib>:"Clear Errors.vi"("error in (no error)"=w445) -> ("error out"=w444:errorcluster)  [unwired: 5 in, 1 out]
          }
        }
        n116 = Compound Arithmetic op=OR ("Opérateur arithmétique")(w416, w421) -> (w420:bool)
        n117 = case shown="Vrai" w420 {
          tunnel: w426 -> [w451 w467]
          tunnel: [w451 refnum<k21> refnum ("task out")] -> w425
          tunnel: [w449 w452] -> w424
          tunnel: [ListeMachineEtats."Rec" ("ListeMachineEtats") w459] -> w423
          tunnel: w408 -> [_ w463]
          tunnel: w406 -> [w449 w458]
          tunnel: w395 -> [w448 w456]
          tunnel: [w448 w455] -> w394
          tunnel: w393 -> [w447 w454]
          tunnel: [w447 w453] -> w392
          frame False {
          }
          frame True {
            n118 = call <vilib>:"DAQmx Stop Task.vi"("task/channels in"=w467, "error in"=w458) -> ("task out"=w466:refnum<k21>, "error out"=w465:errorcluster)  [unwired: 12 in]
            n119 = call <vilib>:"DAQmx Clear Task.vi"("task in"=w466, "error in"=w465) -> ("error out"=w452:errorcluster)  [unwired: 13 in]
            n120 = Equal To 0?(x=w463) -> (x = 0?=w462:bool)
            n121 = call-poly <vilib>:"DAQmx Write.vi"("task/channels in"=w454, "data"=FALSE, "error in"=w456) -> ("task out"=w453:refnum<k21>, "error out"=w455:errorcluster)  [unwired: 10 in, 1 out]
            n122 = Select(t=ListeMachineEtats."InitLect" ("ListeMachineEtats"), s=w462, f=ListeMachineEtats."Processing" ("ListeMachineEtats")) -> (s? t:f=w459:T2)
          }
        }
        n123 = To Double Precision Float(number=w408) -> (double precision float=w414:dbl)
        n124 = Divide(x=w414, y=10.0) -> (x/y=→"Acquisition Time":dbl)
      }
      frame "Processing" {
        w480 = u32 0
        n125 = call "GetFilesPCI.vi"("error in (no error)"=w479, "Test Num :"=w473, "Project :"=w478) -> ("error out"=w476:errorcluster, "NomProjetOut"=w474:string)  [unwired: 3 in]
        n126 = disable-structure shown="Activé" {
          disable-tunnel: w476 -> [w500 w503]
          disable-tunnel: [w499 w501] -> w475
          disable-tunnel: w474 -> [w494 w501]
          disable-tunnel: w473 -> [w498 _]
          disable-tunnel: [w495 w502] -> w472
          frame Disabled {
            n127 = call "MergeFileAutoConfig.vi"("error in (no error)"=w500, "test num"=w498, "ProjetIN"=w494) -> ("error out"=w497:errorcluster, "MergeFileConfigOUT"=w496:T12, "ProjetOUT"=w499:string)  [unwired: 2 in]
            n128 = call "MergeFilesManual.vi"("Error In"=w497, "MergeFileConfINPUT"=w496) -> ("sortie d'erreur"=w495:errorcluster)  [unwired: 5 in]
          }
          frame Enabled {
            n129 = call "BackUpNetworkDisk.vi"("Entrée d'erreur"=w503, "NomProjet"=w501) -> ("error out"=w502:errorcluster)  [unwired: 2 in, 1 out]
          }
        }
        n130 = call "EssaisRealises.vi"("entrée d'erreur (pas d'erreur)"=w472, "WhichPath?"=WhichPath."MeasTDMS", "NomProjet"=w475) -> ("sortie d'erreur"=w485:errorcluster, "InfosFichiers"=w481:string[][])  [unwired: 1 in]
        n131 = property on="Test List" class="ListeMCol (strict)"(error in=w485, "ItemNames"=w481) -> (error out=w484:errorcluster)  [unwired: 1 in, 1 out]
        n132 = Increment(x=w473) -> (x+1=w482:u32)
        n133 = property on="NextTest Num" class="NumNb (strict)"(error in=w484, "Value"=w482) -> (error out=w483:errorcluster)  [unwired: 1 in, 1 out]
      }
      frame "Quit" {
        (unwired) T6 {"Graph2Index"=[], "Graph1Index"=[]} ("GraphIndex")
        w521 = u32 0
        w504 = refnum<k21> refnum ("task out")
        w525 = "" ("NomProjet")
        n134 = call <vilib>:"DAQmx Stop Task.vi"("task/channels in"=w506, "error in"=w507) -> ("task out"=w508:refnum<k21>, "error out"=w509:errorcluster)  [unwired: 12 in]
        n135 = call <vilib>:"DAQmx Stop Task.vi"("task/channels in"=w516, "error in"=w517) -> ("task out"=w519:refnum<k21>, "error out"=w518:errorcluster)  [unwired: 12 in]
        n136 = call <vilib>:"DAQmx Clear Task.vi"("task in"=w508, "error in"=w509) -> ("error out"=w505:errorcluster)  [unwired: 13 in]
        n137 = call <vilib>:"DAQmx Clear Task.vi"("task in"=w519, "error in"=w518) -> ("error out"=w514:errorcluster)  [unwired: 13 in]
        n138 = call <vilib>:"Clear Errors.vi"("error in (no error)"=w514) -> ("error out"=w515:errorcluster)  [unwired: 5 in, 1 out]
        n139 = disable-structure shown="Activé" {
          disable-tunnel: w515 -> [w532 _]
          disable-tunnel: [w531 _] -> w512
          disable-tunnel: w513 -> [w530 _]
          disable-tunnel: [w529 _] -> w510
          frame Enabled {
            n140 = invoke class="VI" method="FA.Fermer"(reference=w530, error in=w532) -> (reference out=w529:refnum<vi>, error out=w531:errorcluster)  [unwired: 1 in, 1 out]
          }
          frame Disabled {
          }
        }
        n141 = Close Reference(reference=w510, error in (no error)=w512) -> (error out=w511:errorcluster)
      }
    }
    "message" <- w77
    "Graph1" <- w42
    "Projet :" <- w52
    n142 = Unbundle By Name(w45) -> ("status"=w49:bool)
    n143 = Select(t=ListeMachineEtats."Quit" ("ListeMachineEtats"), s=w49, f=w48) -> (s? t:f=w46:T2)
    "num iteration" <- w55
  }
  n144 = Unbundle By Name(w25) -> ("ModifConfig"=w24:refnum<vi>, "Bouton Rec"=w23:refnum<vi>, "Bouton Stop"=w22:refnum<vi>, "Bouton Quit"=w21:refnum<vi>, "Test List"=w20:refnum<vi>, "NextTest Num"=w19:refnum<vi>, "message"=w18:refnum<vi>)
  n145 = Close Reference(reference=w24, error in (no error)=w17) -> (error out=w16:errorcluster)
  n146 = Close Reference(reference=w23, error in (no error)=w16) -> (error out=w15:errorcluster)
  n147 = Close Reference(reference=w22, error in (no error)=w15) -> (error out=w14:errorcluster)
  n148 = Close Reference(reference=w21, error in (no error)=w14) -> (error out=w13:errorcluster)
  n149 = Close Reference(reference=w20, error in (no error)=w13) -> (error out=w12:errorcluster)
  n150 = Close Reference(reference=w19, error in (no error)=w12) -> (error out=w11:errorcluster)
  n151 = Close Reference(reference=w18, error in (no error)=w11) -> ()  [unwired: 1 out]
